vi "Name.Create.vi"(10 "PID Number":u16, 11 "PID Name":string) -> (3 "VS Name":string)   [LabVIEW 2019, in "Diagnostics Addon System Explorer.lvlib"]
uses:
  Diagnostics Addon System Explorer.lvlib
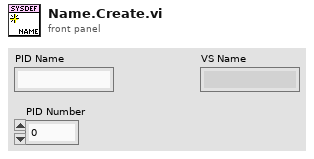
[diagram p1: front panel]
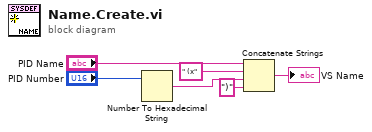
[diagram p0: block diagram]
diagram:
  n1 = Number To Hexadecimal String(2:"PID Number") -> (0:w2:string)  [unwired: 1 in]
  n2 = Concatenate Strings("PID Name", " (x" ("string"), w2, ")" ("string")) -> (→"VS Name":string)
